vi "ConfigureOutputPowerSupply.vi"(0 "VISA resource name":refnum<visa-resource-name>, 1 "Manual Range(0.00)":dbl format="%.2f", 5 "Channel(1: Channel 1)":u16(ring)=1 items=["Channel 1"=1, "Channel 2"=2, "Channel 3"=3], 7 "Function(0:Voltage)":u16(ring) items=["Voltage", "Current"], 9 "Output Enable (T: Enable)":bool=TRUE, 11 "error in (no error)":errorcluster, 12 "Unit(V)":u16(ring) items=["V", "mV", "uV", "kV", "A", "mA", "uA"]) -> (4 "VISA resource name out":refnum<visa-resource-name>, 15 "error out":errorcluster)   [LabVIEW 2009]
doc: "This VI is used to configure voltage or current value for selected channel.\nSelect the channel and output on/off and then set the Voltage or current value as per the selection of the voltage and current."
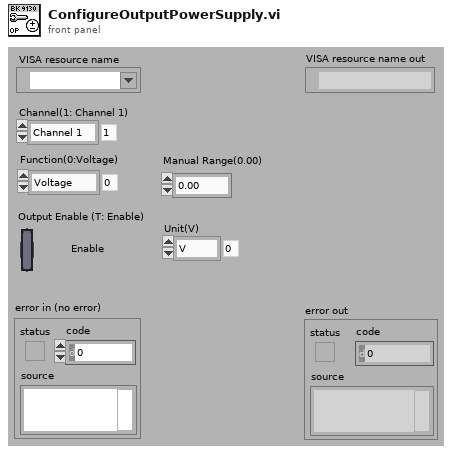
[diagram p1: front panel]
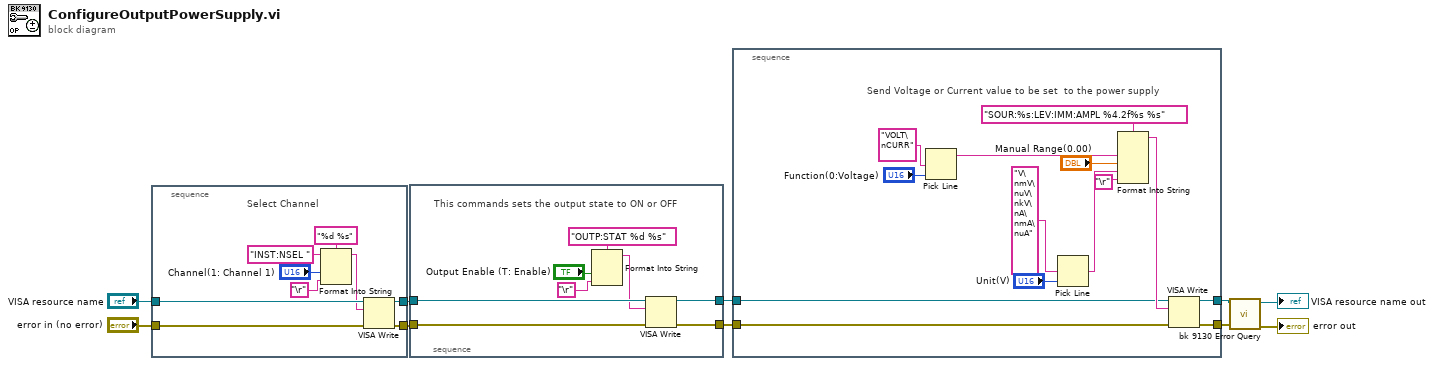
[diagram p0: block diagram]
diagram:
  n1 = stacked-sequence {
    tunnel: [w19] -> w2
    tunnel: [w18] -> w1
    tunnel: "VISA resource name" -> [w14]
    tunnel: "error in (no error)" -> [w13]
    frame #0 {
      # "Select Channel"
      n2 = Format Into String(format string="%d %s", initial string="INST:NSEL ", "Channel(1: Channel 1)", "\r") -> (resulting string=w12:string)  [unwired: 1 in, 1 out]
      n3 = VISA Write(VISA resource name=w14, write buffer=w12, error in (no error)=w13) -> (VISA resource name out=w19:refnum<visa-resource-name>, error out=w18:errorcluster)  [unwired: 1 out]
    }
  }
  n4 = stacked-sequence {
    tunnel: w2 -> [w25]
    tunnel: w1 -> [w24]
    tunnel: [w23] -> w4
    tunnel: [w22] -> w3
    frame #0 {
      # "This commands sets the output state to ON or OFF"
      n5 = Format Into String(format string="OUTP:STAT %d %s", "Output Enable (T: Enable)", "\r") -> (resulting string=w21:string)  [unwired: 2 in, 1 out]
      n6 = VISA Write(VISA resource name=w25, write buffer=w21, error in (no error)=w24) -> (VISA resource name out=w23:refnum<visa-resource-name>, error out=w22:errorcluster)  [unwired: 1 out]
    }
  }
  n7 = stacked-sequence {
    tunnel: [w41] -> w8
    tunnel: [w40] -> w7
    tunnel: w4 -> [w32]
    tunnel: w3 -> [w31]
    frame #0 {
      # "Send Voltage or Current value to be set  to the power supply"
      n8 = Pick Line(multi-line string="VOLT\nCURR" ("format string"), line index="Function(0:Voltage)") -> (output string=w34:string)  [unwired: 1 in]
      n9 = Pick Line(multi-line string="V\nmV\nuV\nkV\nA\nmA\nuA", line index="Unit(V)") -> (output string=w35:string)  [unwired: 1 in]
      n10 = Format Into String(format string="SOUR:%s:LEV:IMM:AMPL %4.2f%s %s", w34, "Manual Range(0.00)", w35, "\r") -> (resulting string=w33:string)  [unwired: 2 in, 1 out]
      n11 = VISA Write(VISA resource name=w32, write buffer=w33, error in (no error)=w31) -> (VISA resource name out=w41:refnum<visa-resource-name>, error out=w40:errorcluster)  [unwired: 1 out]
    }
  }
  n12 = call "bk 9130 Error Query.vi"("error in (no error)"=w7, "VISA resource name"=w8) -> ("error out"=→"error out":errorcluster, "VISA resource name out"=→"VISA resource name out":refnum<visa-resource-name>)  [unwired: 6 in, 2 out]
